vi "New Data (SubVI).vi"(8 "entrée d'erreur (pas d'erreur)":errorcluster, 11 "Refnum VISA en entrée":refnum<visa-resource-name>) -> (0 "sortie d'erreur":errorcluster, 2 "x = y ?":bool, 3 "Refnum VISA en sortie":refnum<visa-resource-name>)   [LabVIEW 2017]
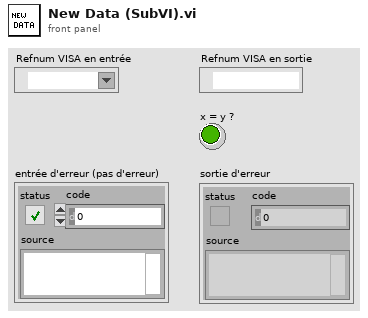
[diagram p1: front panel]
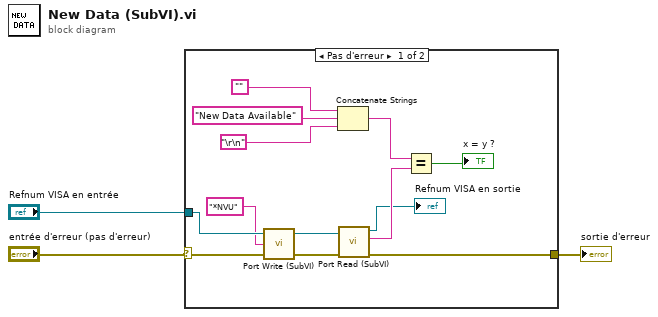
[diagram p0: block diagram]
diagram:
  n1 = case shown="Pas d'erreur" "entrée d'erreur (pas d'erreur)" {
    selector: "entrée d'erreur (pas d'erreur)" -> [w10 w17]
    tunnel: "Refnum VISA en entrée" -> [w16 _]
    tunnel: [w15 w17] -> w2
    frame No Error {
      n2 = call "Port Write (SubVI).vi"("error in"=w10, "write buffer"="*NVU", "VISA Refnum in"=w16) -> ("error out"=w13:errorcluster, "VISA Refnum out"=w12:refnum<visa-resource-name>)  [unwired: 1 in]
      n3 = Concatenate Strings("", "New Data Available", "\r\n") -> (w4:string)
      n4 = call "Port Read (SubVI).vi"("VISA Refnum in"=w12, "error in"=w13) -> ("VISA Refnum out"=→"Refnum VISA en sortie":refnum<visa-resource-name>, "chaîne concaténée"=w14:string, "error out"=w15:errorcluster)  [unwired: 1 out]
      n5 = Equal?(x=w4, y=w14) -> (x = y?=→"x = y ?":bool)
    }
    frame Error {
    }
  }
  "sortie d'erreur" <- w2
